vi "Set configuration chain.vi"(8 "error in (no error)":errorcluster, 9 "class names":string[](array[string]), 10 "configuration":variant[](array[variant]), 11 "ServiceManager in":refnum<class "ServiceManager.lvclass">) -> (0 "error out":errorcluster, 3 "ServiceManager out":refnum<class "ServiceManager.lvclass">)   [LabVIEW 2012, in "ServiceManager.lvclass"]
uses:
  ServiceManager.lvclass
  ServiceManager.lvclass/ServiceManager.ctl
  <vilib>/Distrio/Murmex/Murmex/Murmex.lvclass
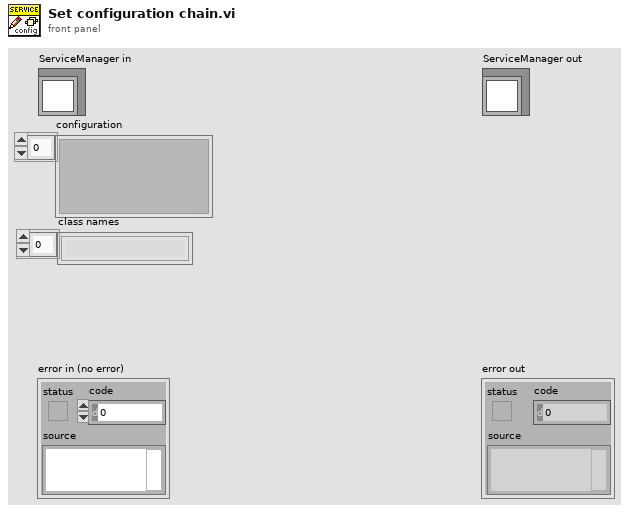
[diagram p1: front panel]
types:
  T1 = typedef "ServiceManager.lvclass/configuration_cluster.ctl" = cluster{"search paths":string[]}
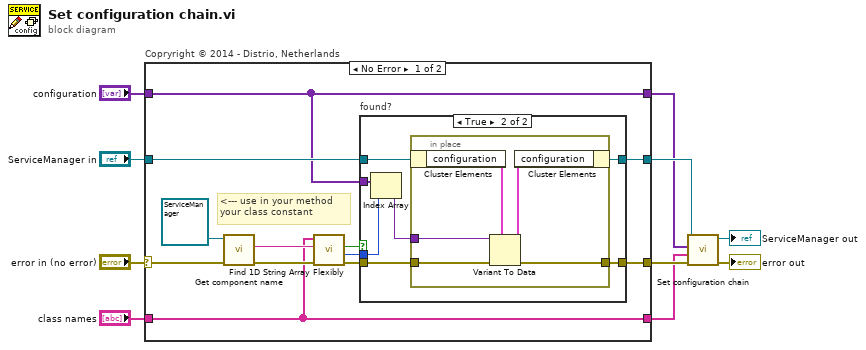
[diagram p0: block diagram]
diagram:
  n1 = case "Copryright © 2014 - Distrio, Netherlands" shown="No Error" "error in (no error)" {
    selector: "error in (no error)" -> [w22 w38]
    tunnel: [w20 w38] -> w5
    tunnel: [w21 w37] -> w4
    tunnel: "ServiceManager in" -> [w14 w37]
    tunnel: "class names" -> [w13 _]
    tunnel: "configuration" -> [w12 _]
    tunnel: [w13 _] -> w2
    tunnel: [w12 _] -> w1
    frame No Error {
      # "<--- use in your method\nyour class constant"
      n2 = call <vilib>:"Get component name.vi"("error in (no error)"=w22, "Murmex in"=refnum<class "ServiceManager.lvclass"> refnum ("ServiceManager in")) -> ("error out"=w19:errorcluster, "component name"=w17:string)  [unwired: 7 in, 1 out]
      n3 = call <vilib>:"Find 1D String Array Flexibly.vi"("error in (no error)"=w19, "element"=w17, "array"=w13) -> ("error out"=w18:errorcluster, "index of element"=w16:i32, "found?"=w15:bool)  [unwired: 6 in]
      n4 = case "found?" shown="True" w15 {
        tunnel: w12 -> [_ w31]
        tunnel: w14 -> [w24 w29]
        tunnel: [w24 w28] -> w21
        tunnel: [w23 w27] -> w20
        tunnel: w18 -> [w23 w26]
        tunnel: w16 -> [_ w25]
        frame False {
        }
        frame True {
          n5 = Index Array(array=w31, index=w25) -> (element=w30:variant)
          n6 = in-place {
            in-place-border: w30 -> [w36]
            in-place-border: w26 -> [w34]
            in-place-border: [w32] -> w27
            n7 = in-place-cluster #1(w29) -> ("configuration"=w35:T1)
            n8 = Variant To Data(error in=w34, type=w35, Variant=w36) -> (data=w33:T1, error out=w32:errorcluster)
            n9 = in-place-cluster #1("configuration"=w33) -> (w28:refnum<class "ServiceManager.lvclass">)
          }
        }
      }
    }
    frame Error {
    }
  }
  n10 = call-parent "Set configuration chain.vi"("error in (no error)"=w5, "class names"=w2, "configuration"=w1, "Murmex in"=w4) -> ("error out"=→"error out":errorcluster, "Murmex out"=→"ServiceManager out":refnum<class "ServiceManager.lvclass">)  [unwired: 6 in]
